vi "gain_atten.vi"() -> ()   [LabVIEW 2014]
doc: "Bode plot ATTEN\nProgramma l'ATF10B per generare un seno con ampiezza e offset scelti\nAcquisiscesia l;inout che la risposta di un circuito\nVaria la frequenza tra FMIN e FMAX e genera il grafico della risposta in funzione della frequenza\nFM & ADL 09-2009, 10/2012\n10/2013: versione per 8.6"
uses:
  <vilib>/DAQmx/read.llb/DAQmx Read (Analog 1D Wfm NChan NSamp).vi
  <vilib>/Instr/_visa.llb/VISA Configure Serial Port (Instr).vi
  <vilib>/DAQmx/create/channels.llb/DAQmx Create Channel (AI-Voltage-Basic).vi
  <vilib>/DAQmx/configure/timing.llb/DAQmx Timing (Sample Clock).vi
  <vilib>/DAQmx/miscellaneous.llb/DAQmx Fill In Error Info.vi
  <vilib>/measure/matone.llb/Extract Single Tone Information 1 Chan.vi
  <vilib>/Utility/file.llb/Write To Spreadsheet File (DBL).vi
  <vilib>/measure/NI_MAPro.lvlib
  <resource>/objmgr/daqmx.rc
panel:
  in  "physical channels":tag="Dev1/ai0"
  in  "Offset (V)":dbl min=-10.0 max=10.0 step=0.05
  in  "Ampiezza (V)":dbl=5.0 min=0.01 max=10.0 step=0.05
  in  "FScala Out (33)":dbl(ring)=5.0 items=["10"=10.0, "5"=5.0, "0.5"=0.5, "0.05"=0.05]
  out "Frequenza":dbl=79999.99999999977 format="%#_1f"
  out "Misura corrente":i16=50
  in  "F_campionamento (Hz)":dbl=1600000.0
  out "Risposta ATF":string="Receive ok\n"
  in  "SALVA I DATI SU FILE":bool=TRUE caption="ON\nOFF"
  out "GAIN":cluster{dbl[], dbl[]}(graph)={[100.0, 114.6163923198291, 131.3691738841298, 150.57060772635268, 172.57859846998727, 197.80336348242318, 226.7150791108317, 259.8526445218818, 297.8337264986509, 341.36627242446053, 391.2617060495962, 448.4500520030617, 513.9972709623069, 589.1251285993726, 675.2339686501547, 773.928814584813, 887.049286400732, 1016.7038901713074, 1165.3093194897099, 1335.6355013658567, 1530.8572262084067, 1754.613324247481, 2011.074491415488, 2305.0210289247834, 2641.9319455669906, 3028.087083553956, 3470.6841714722727, 3977.9729861568703, 4559.40912419038, 5225.830249248129, 5989.658100446539, 6865.130027024227, 7868.564365040478, 9018.664602573064, 10336.868002894698, 11847.745183780671, 13579.45810089571, 15564.28497182944, 17839.221925088234, 20446.6725884641, 23435.238470344968, 26860.624866258106, 30786.679176267957, 35286.58098691841, 40444.206100220625, 46355.68993446913, 53131.219437854656, 60897.086915200794, 69798.04405007385, 79999.99999999977], [0.8699183651397467, 0.8693428764059666, 0.8693392724963684, 0.8696344195702392, 0.8696243231792918, 0.8696458132112024, 0.8696950150183576, 0.8696996889288766, 0.8697088539352634, 0.8697627013159807, 0.8697752866943566, 0.8697155152171341, 0.8698119148361998, 0.8698073086604229, 0.8699283379859623, 0.8699010303023812, 0.8699472670508508, 0.870013712829436, 0.8700179791972786, 0.8700702080788518, 0.8701332929497709, 0.870166248957997, 0.8701775937645315, 0.8701191792031008, 0.8702027921667363, 0.8701371104644144, 0.8701165332193691, 0.8700937194533378, 0.8700235501311662, 0.869903132947068, 0.8697886748460212, 0.8696277782612922, 0.8694308915159261, 0.8692104721806284, 0.8689063902046259, 0.8685643310081156, 0.8682059245150274, 0.8677659532021871, 0.8672780597149495, 0.8667452986917002, 0.8660548540799435, 0.8653427847715575, 0.8645143253798888, 0.8635199670977652, 0.8623129504979143, 0.8608303146920478, 0.8590451502628111, 0.8567592851986922, 0.8539055837210598, 0.850320433606331]}
  out "Vout (bianco) Vin (giallo)":waveform(dbl)[](graph)=[{"t0"=timestamp(3464159597.046872 s since 1904-01-01), "dt"=5.999999999999604e-07, "Y"=array[20000 elements], "attributes"=variant("NI_ChannelName"=variant(string "Dev1/ai1"), "NI_UnitDescription"=variant(string "Volts"))}]
  in  "Numero misure":i16=50
  in  "Freqmax":dbl=80000.0 min=0.0 max=100000.0
  in  "Freqmin":dbl=100.0 min=0.0 max=100000.0
  # "Primo passo: scegliere frequenza di campionamento, fondo scala canali\nSecondo passo: scegliere l'intervallo di frequenza e il numero di misure\nTerzo passo: impostare ampiezza e offset del generatore\nQuarto passo: scegliere se salvare i dati sul file\nQuinto passo: premere la freccia bianca"
  # "Foma d'onda generata Vin(t)"
  # "I Collegamenti"
  # "I due canali di misura (riferiti a terra) sono il CB68 (Vin) e CB33 (Vout).\nLa terra del circuito e quella del generatore DEVONO essere in comune alla terra della scheda (CB29)."
  # "NO\nSI"
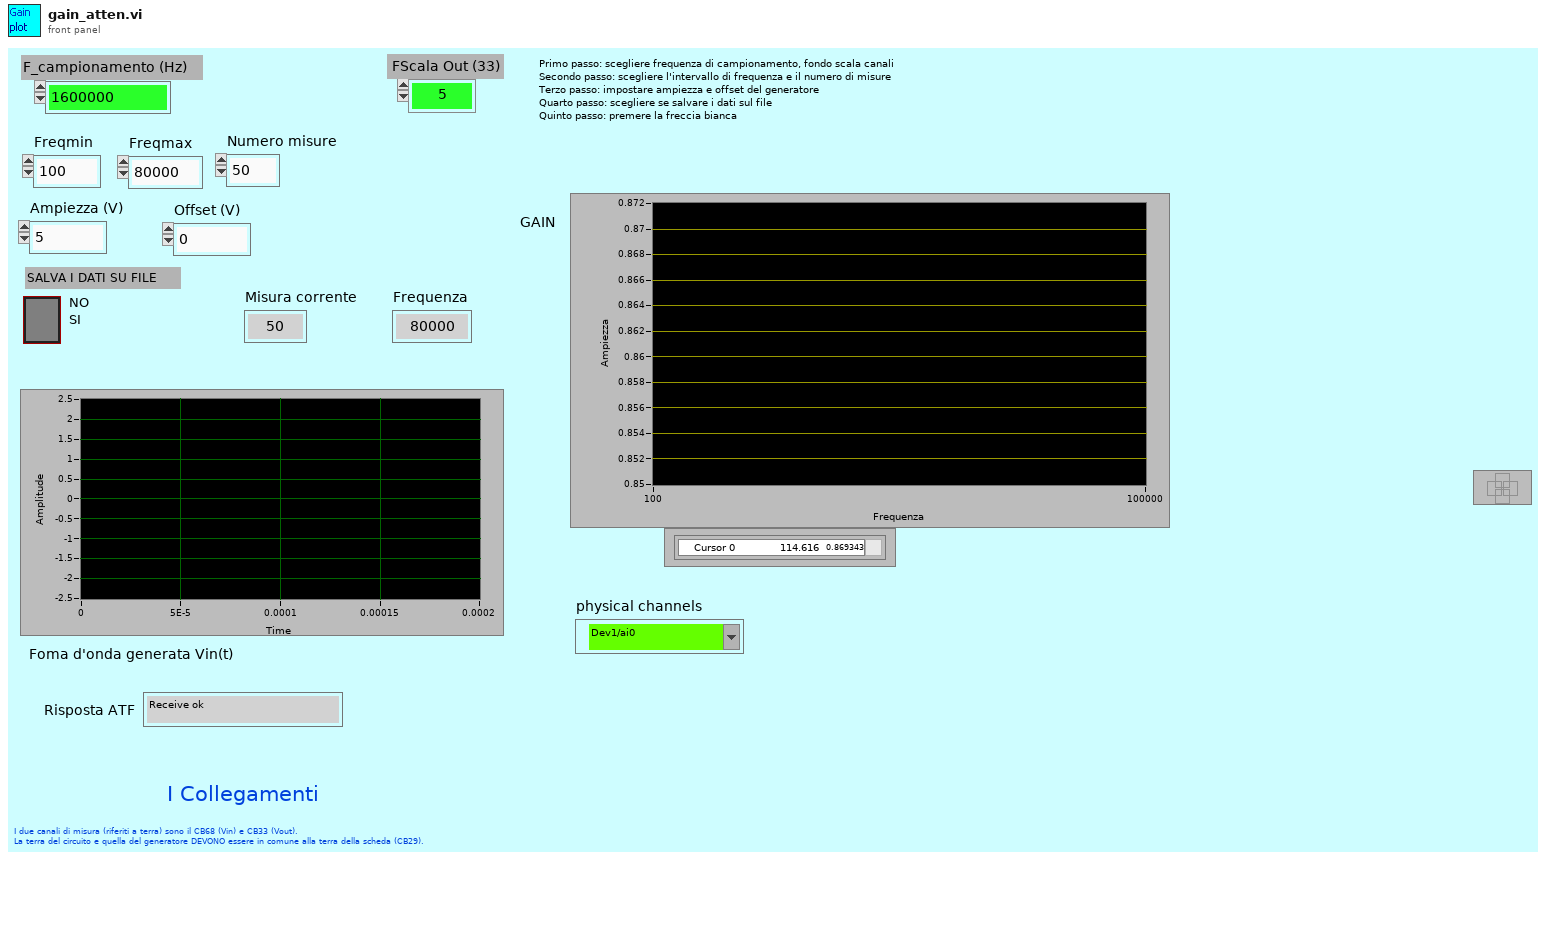
[diagram p1: front panel]
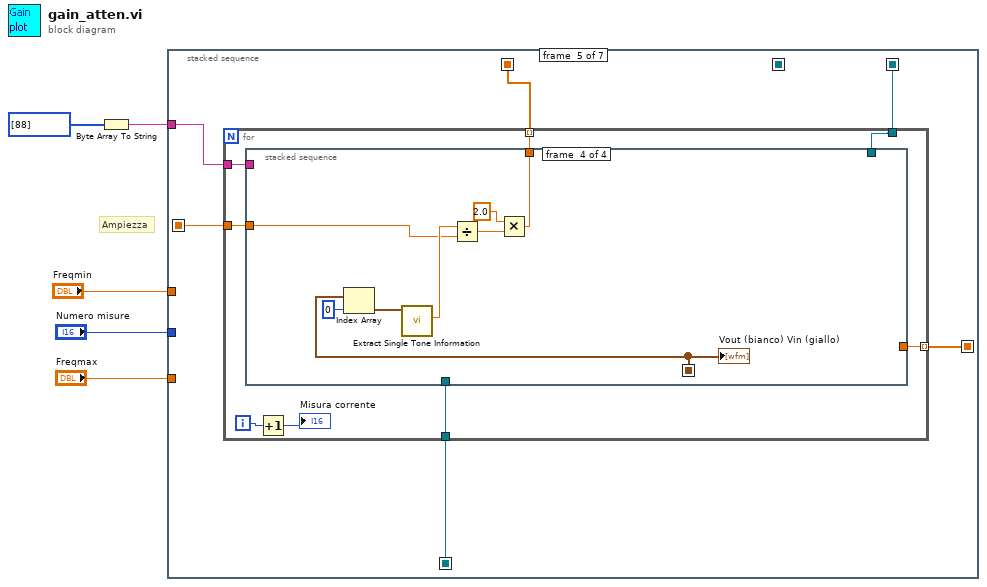
[diagram p0: block diagram]
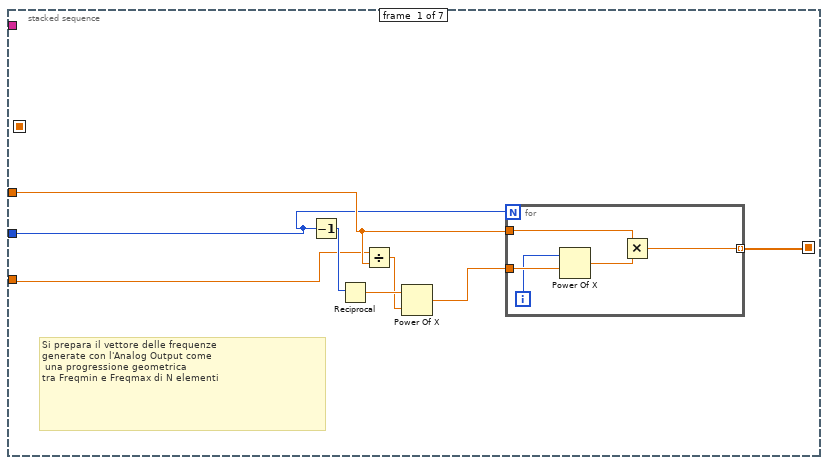
[diagram p2: hidden frame]
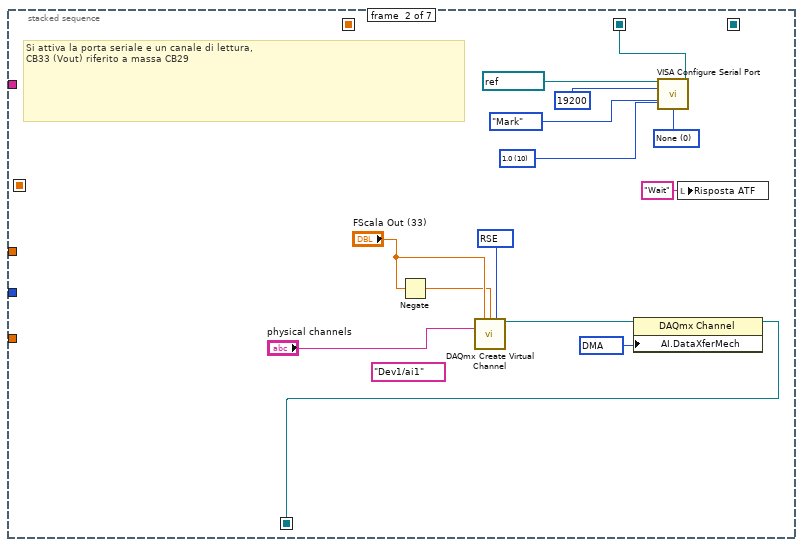
[diagram p3: hidden frame]
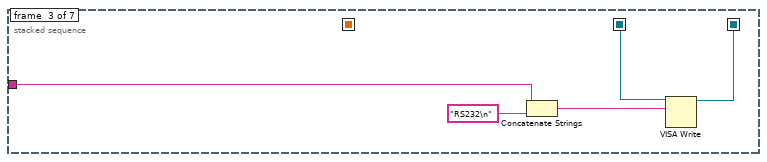
[diagram p4: hidden frame]
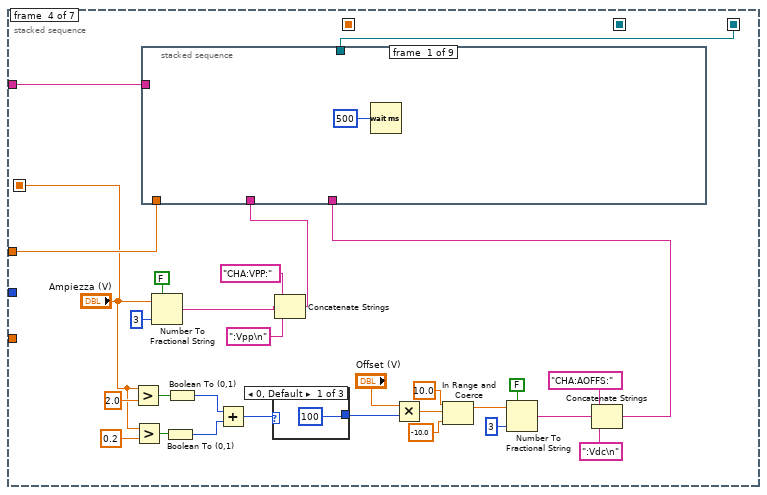
[diagram p5: hidden frame]
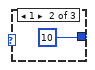
[diagram p6: hidden frame]
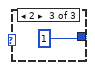
[diagram p7: hidden frame]
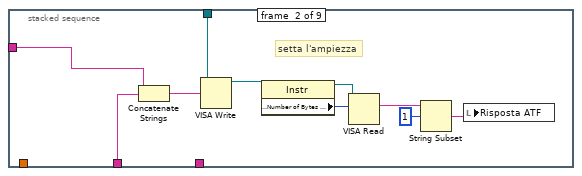
[diagram p8: hidden frame]
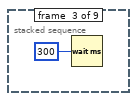
[diagram p9: hidden frame]
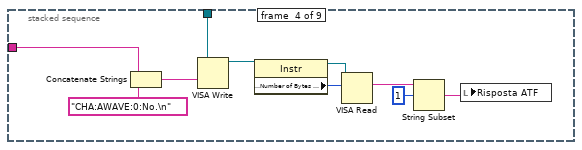
[diagram p10: hidden frame]
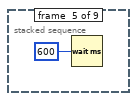
[diagram p11: hidden frame]
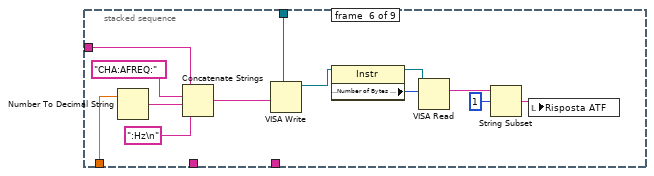
[diagram p12: hidden frame]
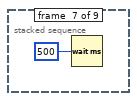
[diagram p13: hidden frame]
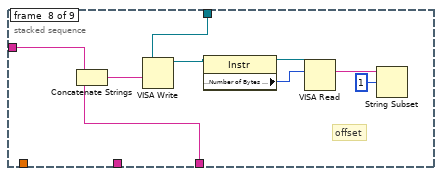
[diagram p14: hidden frame]
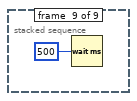
[diagram p15: hidden frame]
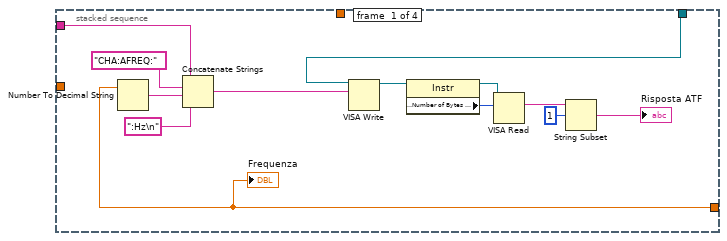
[diagram p16: hidden frame]
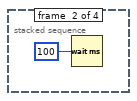
[diagram p17: hidden frame]
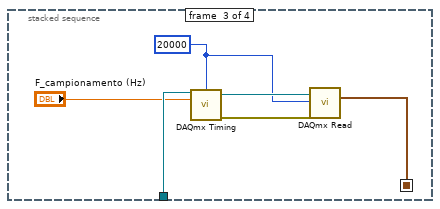
[diagram p18: hidden frame]
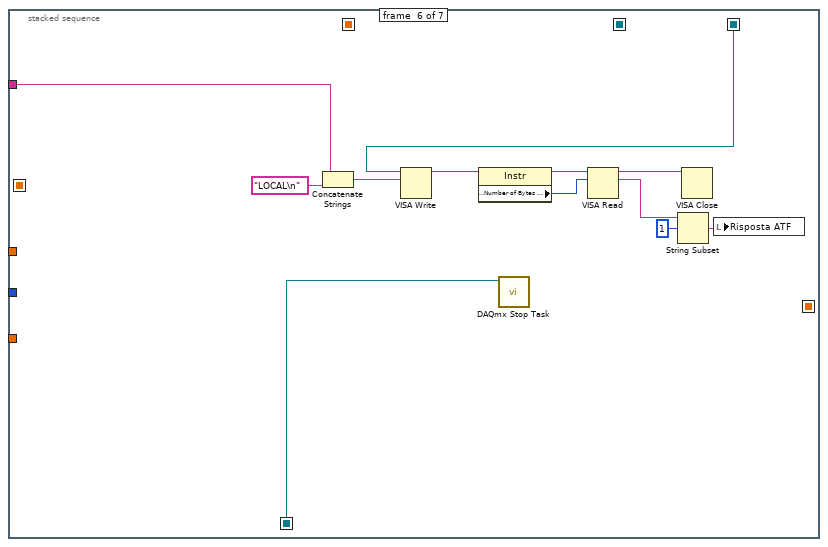
[diagram p19: hidden frame]
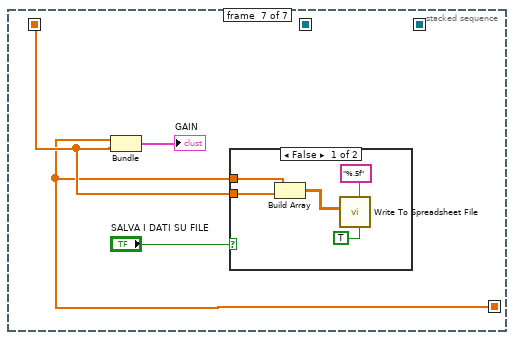
[diagram p20: hidden frame]
diagram:
  # "Ampiezza"
  n1 = Byte Array To String(unsigned byte array=u8[] [88] ("INDIRIZZO")) -> (string=w1:string)
  n2 = stacked-sequence {
    seq-local: [w6 _ _ _ _ _ _] -> [_ _ _ _ w121 _ w171]
    seq-local: [_ w23 _ _ _ _ _] -> [_ _ _ _ w122 w170 _]
    seq-local: [_ _ _ _ w118 _ _] -> [_ _ _ _ _ _ w173]
    seq-local: [_ w28 _ _ _ _ _] -> [_ _ w35 _ _ _ _]
    seq-local: [_ _ w34 _ _ _ _] -> [_ _ _ w65 w120 w167 _]
    seq-local: [_ _ _ "Ampiezza (V)" _ _ _] -> [_ _ _ _ w117 _ _]
    tunnel: "Freqmin" -> [w9 _ _ w64 _ _ _]
    tunnel: "Numero misure" -> [w8 _ _ _ _ _ _]
    tunnel: "Freqmax" -> [w7 _ _ _ _ _ _]
    tunnel: w1 -> [_ _ w33 w66 w119 w159 _]
    frame #0 {
      # "Si prepara il vettore delle frequenze\ngenerate con l'Analog Output come\n una progressione geometrica\ntra Freqmin e Freqmax di N elementi"
      n3 = Decrement(x=w8) -> (x-1=w13:i16)
      n4 = Reciprocal(x=w13) -> (1/x=w12:dbl)
      n5 = Divide(x=w7, y=w9) -> (x/y=w11:dbl)
      n6 = Power Of X(1:w11, 2:w12) -> (0:w10:dbl)
      n7 = for {
        N: w8 -> [_]
        tunnel: w10 -> [w18]
        tunnel: w9 -> [w16]
        tunnel: [w14] -> w6 mode=indexing
        i -> [w17]
        n8 = Power Of X(1:w18, 2:w17) -> (0:w15:dbl)
        n9 = Multiply(x=w16, y=w15) -> (x*y=w14:dbl)
      }
    }
    frame #1 {
      w25 = 10054 items=["DMA"=10054, "Interrupts"=10204, "Programmed I/O"=10264, "USB Bulk"=12590] ("AI.DataXferMech")
      w26 = 10083 items=["default"=-1, "RSE"=10083, "NRSE"=10078, "Differential"=10106, "Pseudodifferential"=12529] ("input terminal configuration")
      (unwired) tag "Dev1/ai1" ("physical channels")
      w30 = u16 10 items=["1.0"=10, "1.5"=15, "2.0"=20] ("stop bits")
      w29 = u16 0 items=["None", "XON/XOFF", "RTS/CTS", "XON/XOFF & RTS/CTS", "DTR/DSR", "XON/XOFF & DTR/DSR"] ("flow control (0:none)")
      # "Si attiva la porta seriale e un canale di lettura,\nCB33 (Vout) riferito a massa CB29"
      n10 = Negate(x="FScala Out (33)") -> (-x=w20:dbl)
      n11 = call-poly <vilib>:"DAQmx Create Virtual Channel.vi"("maximum value"="FScala Out (33)", "minimum value"=w20, "input terminal configuration"=w26, "physical channels"="physical channels") -> ("task out"=w24:refnum<k21>)  [unwired: 5 in, 6 out]
      n12 = property class="DAQmx Channel"(reference=w24, "AI.DataXferMech"=w25) -> (reference out=w23:refnum<k21>)  [unwired: 1 in, 1 out]
      n13 = call-poly "VISA Configure Serial Port"("VISA resource name"=refnum<visa-resource-name> "COM1", "baud rate (9600)"=u32 19200, "parity (0:none)"=enum16{"None", "Odd", "Even", "Mark", "Space"}."Mark" ("parity"), "stop bits (10: 1 bit)"=w30, "flow control (0:none)"=w29) -> ("VISA resource name out"=w28:refnum<visa-resource-name>)  [unwired: 2 in, 8 out]
      n14 = local write "Risposta ATF"("Wait" ("Risposta ATF")) -> ()
    }
    frame #2 {
      n15 = Concatenate Strings(w33, "RS232\n" ("write buffer")) -> (w36:string)
      n16 = VISA Write(VISA resource name=w35, write buffer=w36) -> (VISA resource name out=w34:refnum<visa-resource-name>)  [unwired: 1 in, 2 out]
    }
    frame #3 {
      n17 = Greater?(x="Ampiezza (V)", y=2.0) -> (0:w55:bool)
      n18 = Greater?(x="Ampiezza (V)", y=0.2) -> (0:w54:bool)
      n19 = Number To Fractional String(use system decimal point (T)=FALSE, number="Ampiezza (V)", precision (6)=i16 3) -> (F-format string=w59:string)  [unwired: 1 out]
      n20 = Boolean To (0,1)(Boolean=w54) -> (0, 1=w52:i16)
      n21 = Boolean To (0,1)(Boolean=w55) -> (0, 1=w53:i16)
      n22 = Add(x=w53, y=w52) -> (x+y=w51:i16)
      n23 = case shown="0, Default" w51 {
        tunnel: [100 10 1] -> w50
        frame 0, Default {
        }
        frame 1 {
        }
        frame 2 {
        }
      }
      n24 = Concatenate Strings("CHA:VPP:" ("write buffer"), w59, ":Vpp\n" ("write buffer")) -> (w58:string)
      n25 = Multiply(x="Offset (V)", y=w50) -> (x*y=w48:dbl)
      n26 = In Range and Coerce(upper limit=10.0, x=w48, lower limit=-10.0) -> (coerced(x)=w41:dbl)  [unwired: 1 out]
      n27 = Number To Fractional String(use system decimal point (T)=FALSE, number=w41, precision (6)=i16 3) -> (F-format string=w40:string)  [unwired: 1 out]
      n28 = Concatenate Strings("CHA:AOFFS:" ("write buffer"), w40, ":Vdc\n" ("write buffer")) -> (w39:string)
      n29 = stacked-sequence {
        tunnel: w66 -> [_ w79 _ w89 _ w100 _ w114 _]
        tunnel: w65 -> [_ w78 _ w88 _ w99 _ w113 _]
        tunnel: w64 -> [_ _ _ _ _ w101 _ _ _]
        tunnel: w58 -> [_ w71 _ _ _ _ _ _ _]
        tunnel: w39 -> [_ _ _ _ _ _ _ w107 _]
        frame #0 {
          n30 = Wait (ms)(milliseconds to wait=u32 500 ("millisecond multiple")) -> ()  [unwired: 1 out]
        }
        frame #1 {
          # "setta l'ampiezza"
          n31 = Concatenate Strings(w79, w71) -> (w80:string)
          n32 = VISA Write(VISA resource name=w78, write buffer=w80) -> (VISA resource name out=w73:refnum<visa-resource-name>)  [unwired: 1 in, 2 out]
          n33 = property class="Instr"(reference=w73) -> (reference out=w77:refnum<visa-resource-name>, "Serial Settings:Number of Bytes at Serial Port"=w76:u32)  [unwired: 1 in, 1 out]
          n34 = VISA Read(VISA resource name=w77, byte count=w76) -> (read buffer=w75:string)  [unwired: 1 in, 3 out]
          n35 = String Subset(string=w75, offset (0)=1) -> (substring=w72:string)  [unwired: 1 out]
          n36 = local write "Risposta ATF"(w72) -> ()
        }
        frame #2 {
          n37 = Wait (ms)(milliseconds to wait=u32 300 ("millisecond multiple")) -> ()  [unwired: 1 out]
        }
        frame #3 {
          n38 = Concatenate Strings(w89, "CHA:AWAVE:0:No.\n" ("write buffer")) -> (w91:string)
          n39 = VISA Write(VISA resource name=w88, write buffer=w91) -> (VISA resource name out=w83:refnum<visa-resource-name>)  [unwired: 1 in, 2 out]
          n40 = property class="Instr"(reference=w83) -> (reference out=w87:refnum<visa-resource-name>, "Serial Settings:Number of Bytes at Serial Port"=w86:u32)  [unwired: 1 in, 1 out]
          n41 = VISA Read(VISA resource name=w87, byte count=w86) -> (read buffer=w85:string)  [unwired: 1 in, 3 out]
          n42 = String Subset(string=w85, offset (0)=1) -> (substring=w82:string)  [unwired: 1 out]
          n43 = local write "Risposta ATF"(w82) -> ()
        }
        frame #4 {
          n44 = Wait (ms)(milliseconds to wait=u32 600 ("millisecond multiple")) -> ()  [unwired: 1 out]
        }
        frame #5 {
          n45 = Number To Decimal String(number=w101) -> (decimal integer string=w104:string)  [unwired: 1 out]
          n46 = Concatenate Strings(w100, "CHA:AFREQ:" ("string"), w104, ":Hz\n") -> (w102:string)
          n47 = VISA Write(VISA resource name=w99, write buffer=w102) -> (VISA resource name out=w93:refnum<visa-resource-name>)  [unwired: 1 in, 2 out]
          n48 = property class="Instr"(reference=w93) -> (reference out=w94:refnum<visa-resource-name>, "Serial Settings:Number of Bytes at Serial Port"=w95:u32)  [unwired: 1 in, 1 out]
          n49 = VISA Read(VISA resource name=w94, byte count=w95) -> (read buffer=w96:string)  [unwired: 1 in, 3 out]
          n50 = String Subset(string=w96, offset (0)=1) -> (substring=w98:string)  [unwired: 1 out]
          n51 = local write "Risposta ATF"(w98) -> ()
        }
        frame #6 {
          n52 = Wait (ms)(milliseconds to wait=u32 500 ("millisecond multiple")) -> ()  [unwired: 1 out]
        }
        frame #7 {
          # "offset"
          n53 = Concatenate Strings(w114, w107) -> (w115:string)
          n54 = VISA Write(VISA resource name=w113, write buffer=w115) -> (VISA resource name out=w110:refnum<visa-resource-name>)  [unwired: 1 in, 2 out]
          n55 = property class="Instr"(reference=w110) -> (reference out=w109:refnum<visa-resource-name>, "Serial Settings:Number of Bytes at Serial Port"=w108:u32)  [unwired: 1 in, 1 out]
          n56 = VISA Read(VISA resource name=w109, byte count=w108) -> (read buffer=w112:string)  [unwired: 1 in, 3 out]
          n57 = String Subset(string=w112, offset (0)=1) -> ()  [unwired: 2 out]
        }
        frame #8 {
          n58 = Wait (ms)(milliseconds to wait=u32 500 ("millisecond multiple")) -> ()  [unwired: 1 out]
        }
      }
    }
    frame #4 {
      n59 = for {
        tunnel: w121 -> [w130] mode=indexing
        tunnel: w122 -> [w129]
        tunnel: w120 -> [w123]
        tunnel: w119 -> [w128]
        tunnel: [w127] -> w118 mode=indexing
        tunnel: w117 -> [w124]
        i -> [w126]
        n60 = stacked-sequence {
          seq-local: [_ _ w148 _] -> [_ _ _ w157]
          tunnel: w130 -> [w131 _ _ _]
          tunnel: w129 -> [_ _ w147 _]
          tunnel: w123 -> [w140 _ _ _]
          tunnel: w128 -> [w136 _ _ _]
          tunnel: [_ _ _ w152] -> w127
          tunnel: w124 -> [_ _ _ w153]
          frame #0 {
            n61 = Number To Decimal String(number=w131) -> (decimal integer string=w134:string)  [unwired: 1 out]
            n62 = Concatenate Strings(w136, "CHA:AFREQ:" ("string"), w134, ":Hz\n") -> (w132:string)
            n63 = VISA Write(VISA resource name=w140, write buffer=w132) -> (VISA resource name out=w143:refnum<visa-resource-name>)  [unwired: 1 in, 2 out]
            n64 = property class="Instr"(reference=w143) -> (reference out=w142:refnum<visa-resource-name>, "Serial Settings:Number of Bytes at Serial Port"=w141:u32)  [unwired: 1 in, 1 out]
            n65 = VISA Read(VISA resource name=w142, byte count=w141) -> (read buffer=w139:string)  [unwired: 1 in, 3 out]
            n66 = String Subset(string=w139, offset (0)=1) -> (substring=→"Risposta ATF":string)  [unwired: 1 out]
            "Frequenza" <- w131
          }
          frame #1 {
            n67 = Wait (ms)(milliseconds to wait=u32 100 ("millisecond multiple")) -> ()  [unwired: 1 out]
          }
          frame #2 {
            w145 = 20000 ("samples per channel")
            n68 = call-poly <vilib>:"DAQmx Timing.vi"("task/channels in"=w147, "samples per channel"=w145, "rate"="F_campionamento (Hz)") -> ("task out"=w150:refnum<k21>, "error out"=w149:errorcluster)  [unwired: 4 in, 7 out]
            n69 = call-poly <vilib>:"DAQmx Read.vi"("task/channels in"=w150, "number of samples per channel"=w145, "error in"=w149) -> ("data"=w148:waveform(dbl)[])  [unwired: 12 out]
          }
          frame #3 {
            n70 = Index Array(array=w157, index=0) -> (element=w158:waveform(dbl))
            n71 = call-poly <vilib>:"Extract Single Tone Information.vi"("time signal in"=w158) -> ("detected amplitude"=w154:dbl)  [unwired: 3 in, 7 out]
            n72 = Divide(x=w154, y=w153) -> (x/y=w155:dbl)
            n73 = Multiply(x=2.0, y=w155) -> (x*y=w152:dbl)
            "Vout (bianco) Vin (giallo)" <- w157
          }
        }
        n74 = Increment(x=w126) -> (x+1=→"Misura corrente":i32)
      }
    }
    frame #5 {
      n75 = Concatenate Strings(w159, "LOCAL\n" ("write buffer")) -> (w168:string)
      n76 = VISA Write(VISA resource name=w167, write buffer=w168) -> (VISA resource name out=w166:refnum<visa-resource-name>)  [unwired: 1 in, 2 out]
      n77 = property class="Instr"(reference=w166) -> (reference out=w165:refnum<visa-resource-name>, "Serial Settings:Number of Bytes at Serial Port"=w163:u32)  [unwired: 1 in, 1 out]
      n78 = call <vilib>:"DAQmx Stop Task.vi"("task/channels in"=w170) -> ()  [unwired: 1 in, 14 out]
      n79 = VISA Read(VISA resource name=w165, byte count=w163) -> (VISA resource name out=w164:refnum<visa-resource-name>, read buffer=w161:string)  [unwired: 1 in, 2 out]
      n80 = String Subset(string=w161, offset (0)=1) -> (substring=w160:string)  [unwired: 1 out]
      n81 = VISA Close(VISA resource name=w164) -> ()  [unwired: 1 in, 1 out]
      n82 = local write "Risposta ATF"(w160) -> ()
    }
    frame #6 {
      n83 = Bundle(w171, w173) -> (→"GAIN":cluster{dbl[], dbl[]})  [unwired: 1 out]
      n84 = case shown="False" "SALVA I DATI SU FILE" {
        tunnel: w171 -> [w179 _]
        tunnel: w173 -> [w178 _]
        frame False {
          n85 = Build Array(w179, w178) -> (w177:dbl[][])
          n86 = call-poly <vilib>:"Write To Spreadsheet File.vi"("transpose? (no:F)"=TRUE, "format (%.3f)"="%.5f", "2D data"=w177) -> ()  [unwired: 3 in, 3 out]
        }
        frame True {
        }
      }
    }
  }
